vi "Test high resolution sleep.vi"() -> ()   [LabVIEW 2021]
uses:
  System Time/LabVIEW Time to TAI Time.vi
  Time_CIF_U.lvlib
panel:
  out "Array":cluster{dbl, dbl, dbl, dbl}[](array[cluster])
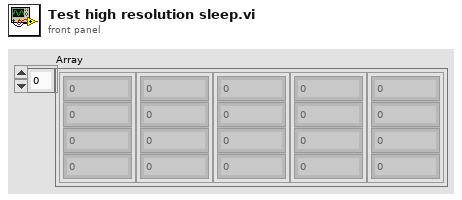
[diagram p1: front panel]
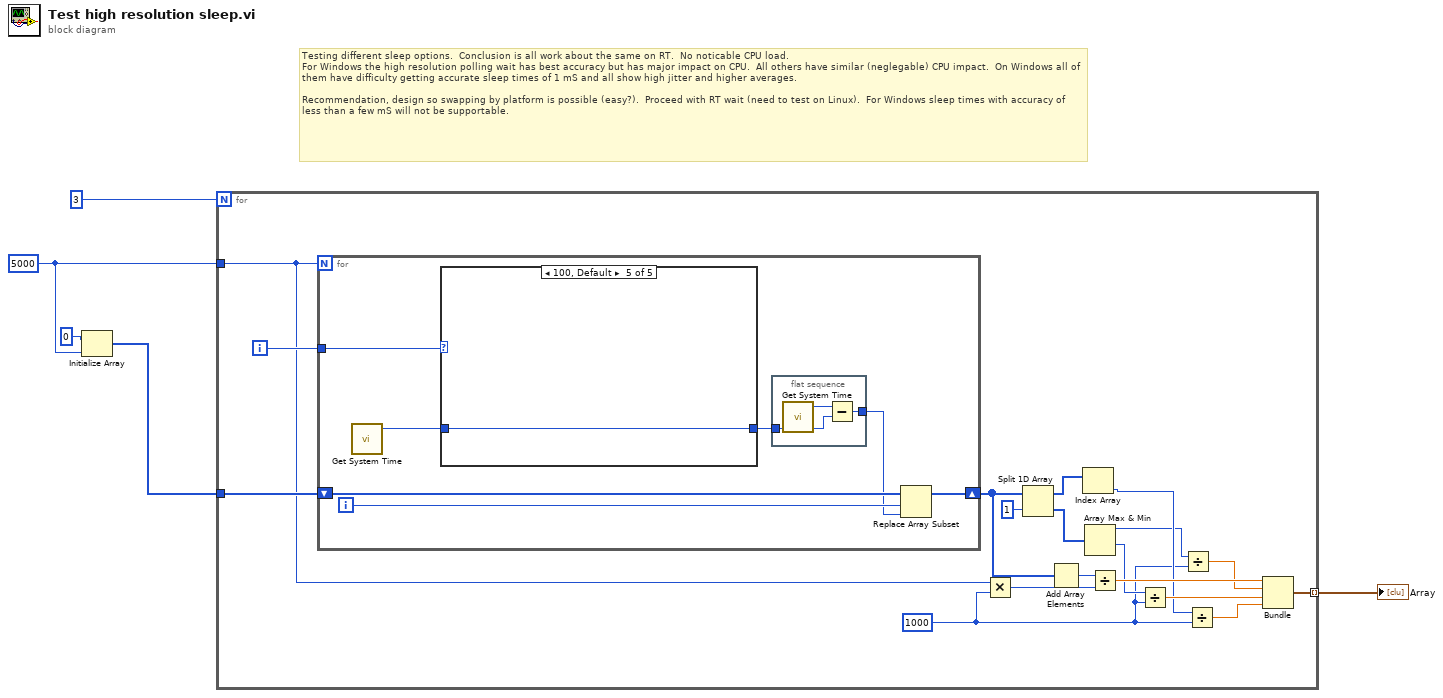
[diagram p0: block diagram]
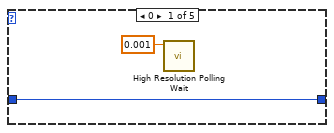
[diagram p2: hidden frame]
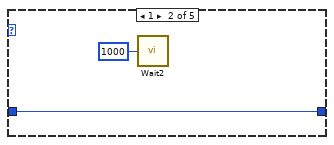
[diagram p3: hidden frame]
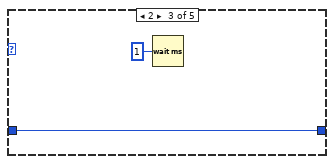
[diagram p4: hidden frame]
diagram:
  w4 = 5000
  # "Testing different sleep options.  Conclusion is all work about the same on RT.  No noticable CPU load.\nFor Windows the high resolution polling wait has best accuracy but has major impact on CPU.  All others have similar (neglegable) CPU impact.  On Windows all of them have difficulty getting accurate sleep times of 1 mS and all show high jitter and higher averages.  \n\nRecommendation, design so swapping by platform is possible (easy?).  Proceed with RT wait (need to test on Linux).  For Windows sleep times with accuracy of less than a few mS will not be supportable."
  n1 = Initialize Array(u64 0, w4) -> (w2:u64[])
  n2 = for {
    N: 3 -> [_]
    tunnel: w4 -> [w8]
    tunnel: w2 -> [w22]
    tunnel: [w21] -> w1 mode=indexing
    i -> [w23]
    w6 = u64 1000 ("y")
    n3 = for {
      N: w8 -> [_]
      tunnel: w23 -> [w30]
      shift-right: [w28] -> w17
      shift-left: w22 -> [w29]
      i -> [w27]
      n4 = call "Get System Time.vi"() -> ("Time (ns)"=w25:i64)  [unwired: 5 in]
      n5 = case shown="100, Default" w30 {
        tunnel: w25 -> [w34 w36 w38 w40 w41]
        tunnel: [w34 w36 w38 w40 w41] -> w24
        frame 0 {
          n6 = call <vilib>:"High Resolution Polling Wait.vi"("seconds to wait"=0.001) -> ()  [unwired: 10 in, 1 out]
        }
        frame 1 {
          n7 = call "Wait2"("Count(uSec)"=u32 1000) -> ()  [unwired: 1 out]
        }
        frame 2 {
          n8 = Wait (ms)(milliseconds to wait=u32 1) -> ()  [unwired: 1 out]
        }
        frame 3 {
        }
        frame 100, Default {
        }
      }
      n9 = flat-sequence {
        tunnel: [w32] -> w26
        tunnel: w24 -> [w31]
        frame #0 {
          n10 = call "Get System Time.vi"() -> ("Time (ns)"=w33:i64)  [unwired: 5 in]
          n11 = Subtract(x=w33, y=w31) -> (x-y=w32:i64)
        }
      }
      n12 = Replace Array Subset(array=w29, new element=w26, index=w27) -> (w28:u64[])
    }
    n13 = Multiply(x=w8, y=w6) -> (x*y=w7:u64)
    n14 = Split 1D Array(array=w17, index=1) -> (first subarray=w19:u64[], second subarray=w18:u64[])
    n15 = Add Array Elements(numeric array=w17) -> (sum=w16:u64)
    n16 = Index Array(array=w19) -> (element=w12:u64)  [unwired: 1 in]
    n17 = Array Max & Min(array=w18) -> (max value=w10:u64, min value=w14:u64)  [unwired: 2 out]
    n18 = Divide(x=w16, y=w7) -> (x/y=w15:dbl)
    n19 = Divide(x=w14, y=w6) -> (x/y=w13:dbl)
    n20 = Divide(x=w10, y=w6) -> (x/y=w9:dbl)
    n21 = Divide(x=w12, y=w6) -> (x/y=w11:dbl)
    n22 = Bundle(w15, w9, w13, w11) -> (w21:cluster{dbl, dbl, dbl, dbl})  [unwired: 1 in]
  }
  "Array" <- w1
